vi "Laser Controller.vi"() -> ()   [LabVIEW 2022 SP3]
uses:
  <vilib>/MakerHub/LINX/Public/Peripherals/PWM/PWM Set Duty Cycle 1 Chan.vi
  <vilib>/MakerHub/LINX/Public/Peripherals/Digital/Digital Read 1 Chan.vi
  <vilib>/MakerHub/LINX/Public/Peripherals/Digital/Digital Read N Chans.vi
  <vilib>/MakerHub/LINX/Private/Local IO/LinxDigitalRead.vi
  <vilib>/MakerHub/LINX/Public/Utilities/Check Channel.vi
  <vilib>/MakerHub/LINX/Public/Utilities/Open Serial.vi
  <vilib>/MakerHub/LINX/Public/Peripherals/PWM/PWM Set Duty Cycle N Chans.vi
  <vilib>/MakerHub/LINX/Private/Utilties/Generate Error.vi
  <vilib>/MakerHub/LINX/LMH-LINX.lvlib
panel:
  out "Trigger Pressed":bool
  out "Recovery Rate":dbl
  out "Drain Rate":dbl
  out "Overheating":bool
  out "Energy":dbl(slide) scale=0.0..100.0
  in  "Recovery Rate":dbl
  in  "Drain Rate":dbl
  in  "Trigger Pin":u8=3
  in  "Laser Pin":u8=6
  in  "Stop Button":bool
  in  "Serial Port":refnum<visa-resource-name>="N/A"
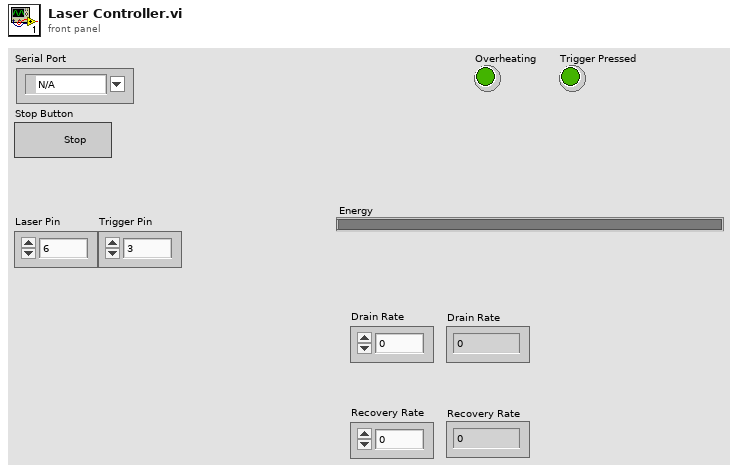
[diagram p1: front panel]
types:
  T1 = typedef "LMH-LINX.lvlib/LINX Ref.ctl" = cluster{"IO":T2, "Interface":T3, "LINX Device Config":T4}
  T2 = typedef "LMH-LINX.lvlib/Platform.ctl" = enum16{"Remote", "Local"}
  T3 = typedef "LMH-LINX.lvlib/Interface.ctl" = enum16{"Serial", "TCP"}
  T4 = typedef "LMH-LINX.lvlib/Device.lvlib/LINX Device Config.ctl" = cluster{"Interface":T3, "COM Port":refnum<visa-resource-name>, "TCP Configuration":T5, "Device Family":u8, "Device ID":u8, "Device Name":string, "TCP Ref":refnum<k5>, "Channels":T6}
  T5 = typedef "LMH-LINX.lvlib/Device.lvlib/TCP Config.ctl" = cluster{"IP Address":string, "Port":u16}
  T6 = typedef "LMH-LINX.lvlib/Channels.ctl" = cluster{"DI":u8[], "DO":u8[], "AI":u8[], "AO":u8[], "PWM":u8[], "QE":u8[], "UART":u8[], "I2C 2":u8[], "SPI":u8[], "CAN":u8[], "Servo":u8[], "AI Ref (V)":dbl, "AI Resolution (Bits)":u8, "AO Ref (V)":dbl, "AO Resolution (Bits)":u8}
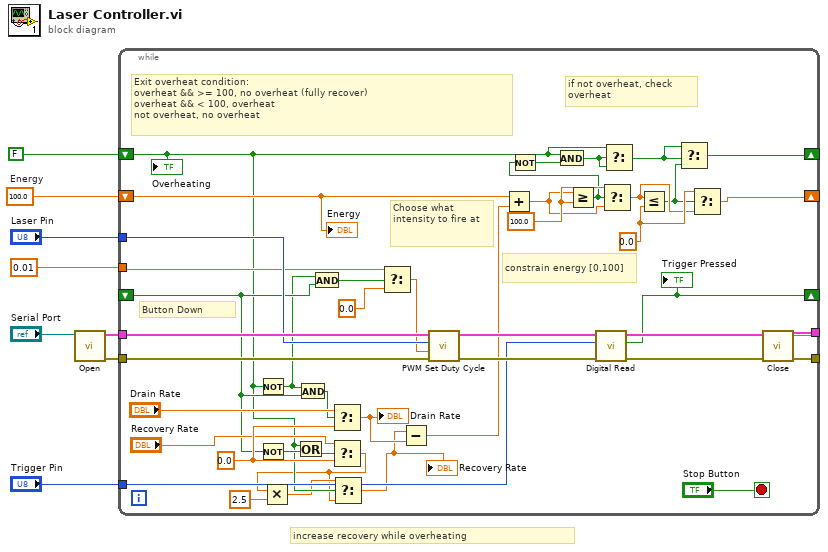
[diagram p0: block diagram]
diagram:
  w2 = 100.0  # Energy
  # "increase recovery while overheating"
  n1 = call-poly <vilib>:"Open.vi"("Serial Port"="Serial Port") -> ("Error Out"=w9:errorcluster, "LINX Resource"=w10:T1)  [unwired: 8 in, 1 out]
  n2 = while {
    tunnel: w10 -> [w47]
    tunnel: w9 -> [w46]
    tunnel: "Laser Pin" -> [w43]
    tunnel: "Trigger Pin" -> [w42]
    tunnel: [w49] -> w5
    tunnel: [w48] -> w4
    shift-right: [w41] -> _
    shift-left: _ -> [w24]
    tunnel: 0.01 -> [w40]
    shift-right: [w33] -> _
    shift-left: w2 -> [w30]
    shift-right: [w22] -> _
    shift-left: FALSE -> [w14]
    stop <- "Stop Button" stop-if-true
    w32 = 0.0 ("y")
    w35 = 100.0 ("y")
    w50 = 0.0
    # "if not overheat, check overheat"
    # "Exit overheat condition:\noverheat && >= 100, no overheat (fully recover)\noverheat && < 100, overheat\nnot overheat, no overheat"
    # "Button Down"
    # "Choose what intensity to fire at"
    # "constrain energy [0,100]"
    n3 = Not(x=w14) -> (.not. x?=w17:bool)
    n4 = Not(x=w24) -> (.not. x?=w28:bool)
    n5 = Or(x=w14, y=w28) -> (x .or. y?=w16:bool)
    n6 = And(x=w17, y=w24) -> (x .and. y?=w25:bool)
    n7 = And(x=w17, y=w24) -> (x .and. y?=w29:bool)
    n8 = Select(t="Drain Rate", s=w25, f=w50) -> (s? t:f=w37:dbl)
    "Drain Rate" <- w37
    n9 = Select(t="Recovery Rate", s=w16, f=w50) -> (s? t:f=w12:dbl)
    n10 = Multiply(x=w12, y=2.5) -> (x*y=w13:dbl)
    n11 = Select(t=w13, s=w14, f=w12) -> (s? t:f=w15:dbl)
    "Recovery Rate" <- w15
    n12 = Select(t=w40, s=w29, f=0.0) -> (s? t:f=w38:dbl)
    n13 = Subtract(x=w15, y=w37) -> (x-y=w36:dbl)
    n14 = call-poly <vilib>:"PWM Set Duty Cycle.vi"("Error In"=w46, "Duty Cycle (0-1)"=w38, "PWM Channel"=w43, "LINX Resource"=w47) -> ("Error Out"=w45:errorcluster, "LINX Resource"=w44:T1)  [unwired: 6 in]
    n15 = Add(x=w30, y=w36) -> (x+y=w34:dbl)
    n16 = Greater Or Equal?(x=w34, y=w35) -> (x >= y?=w21:bool)
    n17 = Not(x=w21) -> (.not. x?=w20:bool)
    n18 = And(x=w14, y=w20) -> (x .and. y?=w18:bool)
    n19 = call-poly <vilib>:"Digital Read.vi"("Error In"=w45, "DI Channel"=w42, "LINX Resource"=w44) -> ("Error Out"=w48:errorcluster, "DI Value"=w41:bool, "LINX Resource"=w49:T1)  [unwired: 6 in]
    "Trigger Pressed" <- w41
    n20 = Select(t=w35, s=w21, f=w34) -> (s? t:f=w31:dbl)
    n21 = Select(t=w14, s=w18, f=w18) -> (s? t:f=w19:bool)
    n22 = Less Or Equal?(x=w31, y=w32) -> (x <= y?=w23:bool)
    n23 = Select(t=w19, s=w19, f=w23) -> (s? t:f=w22:bool)
    n24 = Select(t=w32, s=w23, f=w31) -> (s? t:f=w33:dbl)
    "Energy" <- w30
    "Overheating" <- w14
  }
  n25 = call <vilib>:"Close.vi"("Error In"=w4, "LINX Resource"=w5) -> ()  [unwired: 9 in, 1 out]
